vi "Rec Fetch Binary Data (R).vi"(6 "error in (no error)":errorcluster, 7 "type":variant, 8 "column index":variant, 9 "recordset reference":T1) -> (0 "error out":errorcluster, 1 "data":variant, 3 "recordset reference out":T1)   [LabVIEW 2020, in "NI_Database_API.lvlib"]
doc: "Retrieves the data located at the <B>column index</B> of the current record in the recordset identified by the <B>recordset reference</B>. The <B>column index</B> can be either the zero-indexed position of the column in the recordset or the name of the column. Wire data to the <B>type</B> input to determine the polymorphic instance to use or manually select the instance."
uses:
  <vilib>/addons/database/NI_Database_API.lvlib
  <vilib>/addons/database/Recordset.llb/Rec ObjectReference.ctl
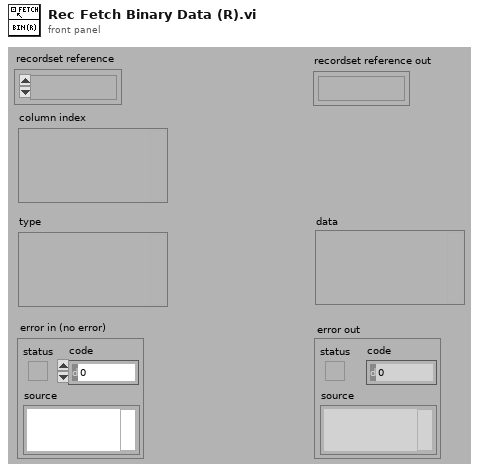
[diagram p1: front panel]
types:
  T1 = typedef "NI_Database_API.lvlib/Rec ObjectReference.ctl" = refnum<k1>
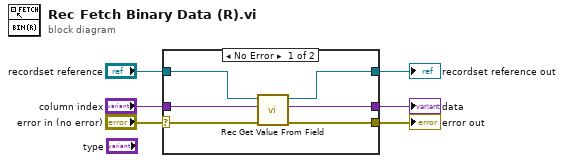
[diagram p0: block diagram]
diagram:
  n1 = case shown="No Error" "error in (no error)" {
    selector: "error in (no error)" -> [w7 w14]
    tunnel: "recordset reference" -> [w12 w13]
    tunnel: [w11 w13] -> w5
    tunnel: [w10 w14] -> w4
    tunnel: "column index" -> [w9 _]
    tunnel: [w8 _] -> w2
    frame No Error {
      n2 = call <vilib>:"Rec Get Value From Field.vi"("error in (no error)"=w7, "column index"=w9, "recordset reference"=w12) -> ("error out"=w10:errorcluster, "value"=w8:variant, "recordset reference out"=w11:T1)  [unwired: 4 in]
    }
    frame Error {
    }
  }
  "data" <- w2
  "error out" <- w4
  "recordset reference out" <- w5
